vi "LVPortConvertObjectMapDataValueToWaveform.vi"(10 "Numbers Vector":variant, 11 "Waveform":variant) -> (3 "Data Value out":variant)   [LabVIEW 2017]
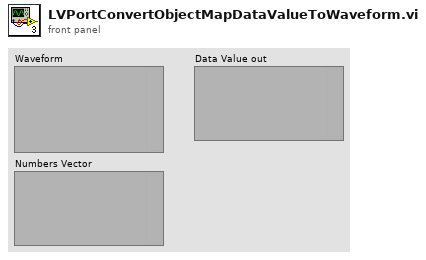
[diagram p1: front panel]
types:
  T1 = typedef "LVPortObjectMapDataTypeEnum.ctl" = enum16{"NotAMatlabType", "Real", "Complex", "String", "Boolean"}
  T2 = typedef "LVPortObjectMapContainerTypeEnum.ctl" = enum16{"Numeric Value", "Numeric Array", "Waveform"}
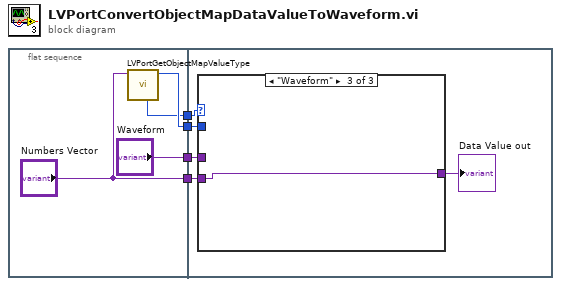
[diagram p0: block diagram]
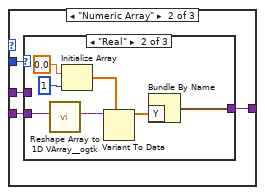
[diagram p3: hidden frame]
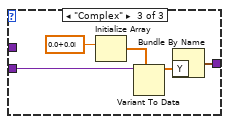
[diagram p5: hidden frame]
diagram:
  n1 = flat-sequence {
    tunnel: ["Waveform"] -> w4
    tunnel: [w6] -> w3
    tunnel: ["Numbers Vector"] -> w2
    tunnel: [w5] -> w1
    tunnel: w4 -> [w12]
    tunnel: w3 -> [w11]
    tunnel: w2 -> [w10]
    tunnel: w1 -> [w9]
    frame #0 {
      n2 = call "LVPortGetObjectMapValueType.vi"("Value"="Numbers Vector") -> ("MatlabType"=w6:T1, "Container Type (Labview Value type)"=w5:T2)  [unwired: 6 in, 3 out]
    }
    frame #1 {
      n3 = case shown="\"Waveform\"" w9 {
        tunnel: [w14 w18 w32] -> w13
        tunnel: w12 -> [w14 w17 _]
        tunnel: w11 -> [_ w16 _]
        tunnel: w10 -> [_ w15 w32]
        frame Default {
        }
        frame "Numeric Array" {
          n4 = case shown="\"Real\"" w16 {
            tunnel: w15 -> [_ w21 w31]
            tunnel: [w19 w23 w27] -> w18
            tunnel: w17 -> [w19 _ _]
            frame Default {
            }
            frame "Real" {
              n5 = call <userlib>:"Reshape Array to 1D VArray__ogtk.vi"("MultiD Array"=w21) -> ("1D VArray"=w20:variant)  [unwired: 8 in, 2 out]
              n6 = Initialize Array(0.0, 1 ("dimension size")) -> (w25:dbl[])
              n7 = Variant To Data(type=w25, Variant=w20) -> (data=w24:dbl[])  [unwired: 1 in, 1 out]
              n8 = Bundle By Name("Y"=w24) -> (w23:waveform(dbl))  [unwired: 1 in]
            }
            frame "Complex" {
              n9 = Initialize Array(cdb 0.0+0.0i) -> (w29:cdb[])  [unwired: 1 in]
              n10 = Variant To Data(type=w29, Variant=w31) -> (data=w28:cdb[])  [unwired: 1 in, 1 out]
              n11 = Bundle By Name("Y"=w28) -> (w27:waveform(cdb))  [unwired: 1 in]
            }
          }
        }
        frame "Waveform" {
        }
      }
      "Data Value out" <- w13
    }
  }
